vi "Fill_State_Controller_run.vi"(2 "error in (no error)":errorcluster) -> (0 "error out":errorcluster)   [LabVIEW 2013]
uses:
  My Computer/Controls/Swimbladder Tuning Parameters.ctl
  My Computer/Controls/Advanced Swimbladder Indicators.ctl
panel:
  out "Motor Power [-]":dbl
  # "maybey implement a security upper kimit"
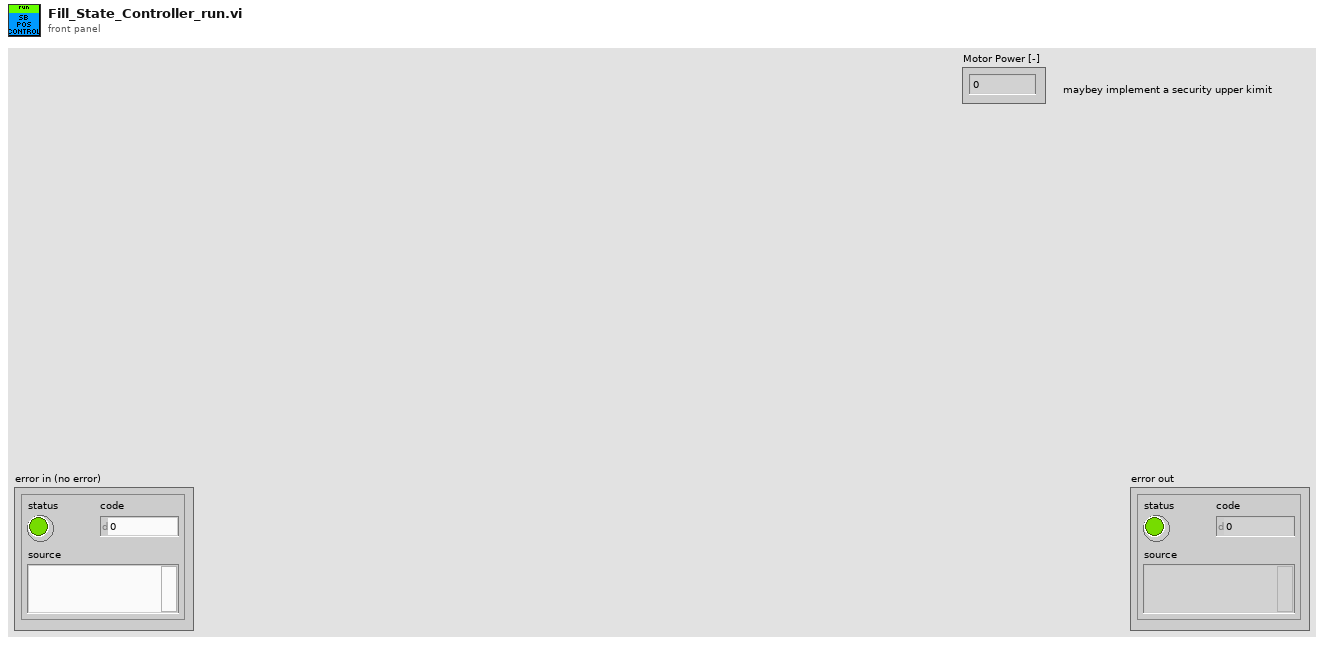
[diagram p1: front panel]
types:
  T1 = typedef "Swimbladder Tuning Parameters.ctl" = cluster{"Excessive_Depth_Deviation_Trigger":dbl, "Neutral Buoancy_x":dbl, "Ti_Depth_Control":dbl, "kp_Depth_Control":dbl, "Integrator enabled range Depth":dbl, "Integrator_enable_Range_Motor":dbl, "kp_Motor":dbl, "Ti_Motor":dbl}
  T2 = typedef "Advanced Swimbladder Indicators.ctl" = cluster{"P_ref [Pa]":dbl, "X_Actual [m]":dbl, "Motor Current[A]":dbl}
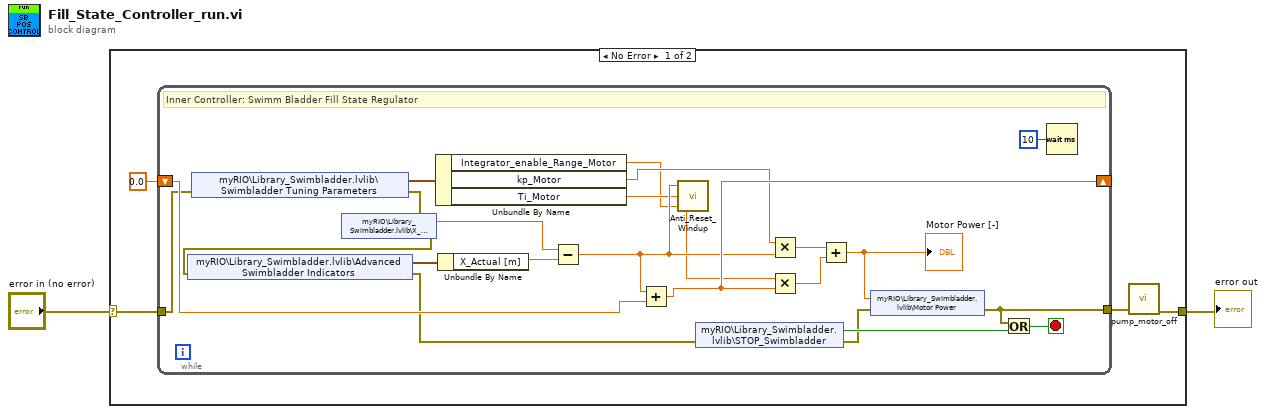
[diagram p0: block diagram]
diagram:
  n1 = case shown="No Error" "error in (no error)" {
    selector: "error in (no error)" -> [w3 w30]
    tunnel: [w4 w30] -> w2
    frame No Error {
      n2 = while {
        tunnel: w3 -> [w11]
        tunnel: [w23] -> w5
        shift-right: [w29] -> _
        shift-left: 0.0 ("Numeric Control in") -> [w28]
        stop <- w24 stop-if-true
        # "Inner Controller: Swimm Bladder Fill State Regulator"
        n3 = shared-variable "myRIO\\Library_Swimbladder.lvlib\\Swimbladder Tuning Parameters"(error in=w11) -> (w18:T1, error out=w7:errorcluster)
        n4 = shared-variable "myRIO\\Library_Swimbladder.lvlib\\X_desired"(error in=w7) -> (w9:dbl, error out=w8:errorcluster)
        n5 = shared-variable "myRIO\\Library_Swimbladder.lvlib\\Advanced Swimbladder Indicators"(error in=w8) -> (w14:T2, error out=w12:errorcluster)
        n6 = Unbundle By Name(w18) -> ("Integrator_enable_Range_Motor"=w15:dbl, "kp_Motor"=w17:dbl, "Ti_Motor"=w16:dbl)
        n7 = Unbundle By Name(w14) -> ("X_Actual [m]"=w13:dbl)
        n8 = Subtract(x=w9, y=w13) -> (x-y=w21:dbl)
        n9 = Add(x=w21, y=w28) -> (x+y=w29:dbl)
        n10 = call "Anti_Reset_Windup.vi"("Integrator enabled range"=w15, "Ti_enabled_in"=w16, "actuall error"=w21) -> ("Ti_out"=w20:dbl)  [unwired: 1 in]
        n11 = shared-variable "myRIO\\Library_Swimbladder.lvlib\\STOP_Swimbladder"(error in=w12) -> (w25:bool, error out=w22:errorcluster)
        n12 = Multiply(x=w17, y=w21) -> (x*y=w26:dbl)
        n13 = Multiply(x=w20, y=w29) -> (x*y=w27:dbl)
        n14 = Add(x=w26, y=w27) -> (x+y=w19:dbl)
        "Motor Power [-]" <- w19
        n15 = shared-variable "myRIO\\Library_Swimbladder.lvlib\\Motor Power"(w19, error in=w22) -> (error out=w23:errorcluster)
        n16 = Or(x=w23, y=w25) -> (x .or. y?=w24:bool)
        n17 = Wait (ms)(milliseconds to wait=u32 10) -> ()  [unwired: 1 out]
      }
      n18 = call "pump_motor_off.vi"("error in (no error)"=w5) -> ("error out"=w4:errorcluster)  [unwired: 10 in]
    }
    frame Error {
    }
  }
  "error out" <- w2
